vi "Fitz9 PID Control.vi"(7 "Pressure Controls":T2 {"output range"."output low" format="%.2f"; "output range"."output high" format="%.2f"; "PID gains"."derivative time (Td, min)" format="%.6f"; "PID gains"."integral time (Ti, min)" format="%.5f"; "PID gains"."proportional gain (Kc)" format="%.3f"; "Phi" scale=0.0..1.5; "Des P drop" scale=0.0..6.0}, 8 "Error In":errorcluster, 10 "Set Point Array":dbl[](array[numeric])) -> (0 "Error Out":errorcluster, 2 "Set Point Array out":dbl[](array[numeric]), 5 "Pressure Indicators":T1)   [LabVIEW 2013]
doc: "This sub-VI controls the air and fuel mass flow controllers for the Fitz9 burner. This burner has one air\nflow controller, and three fuel flow controllers, all with their own set points."
uses:
  Controls/pressure_control_cluster.ctl
  Controls/run_mode_enum.ctl
  Controls/Fitz9_pressure_indicator_cluster.ctl
  <vilib>/DAQmx/read.llb/DAQmx Read (Analog DBL 1Chan 1Samp).vi
  <vilib>/DAQmx/write.llb/DAQmx Write (Analog DBL 1Chan 1Samp).vi
  <vilib>/addons/control/pid/pid.llb/PID (DBL).vi
  <vilib>/DAQmx/miscellaneous.llb/DAQmx Fill In Error Info.vi
  <vilib>/addons/control/pid/NI_PID_pid.lvlib
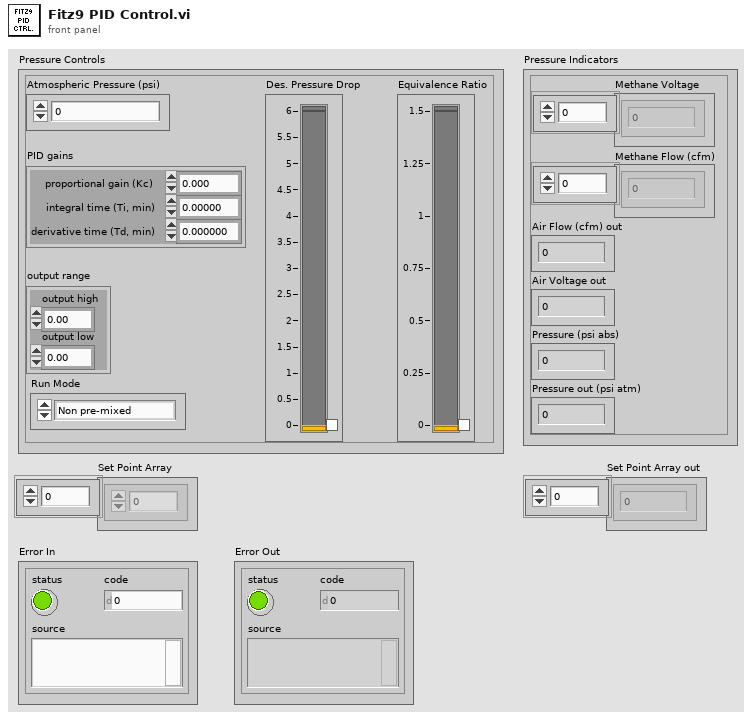
[diagram p1: front panel]
types:
  T1 = typedef "Fitz9_pressure_indicator_cluster.ctl" = cluster{"Methane Voltage":dbl[], "Methane Flow (cfm)":dbl[], "Air Flow (cfm) out":dbl, "Air Voltage out":dbl, "Pressure (psi abs)":dbl, "Pressure out (psi atm)":dbl}
  T2 = typedef "pressure_control_cluster.ctl" = cluster{"Atm Press":dbl, "Des P drop":dbl, "Phi":dbl, "PID gains":cluster{"proportional gain (Kc)":dbl, "integral time (Ti, min)":dbl, "derivative time (Td, min)":dbl}, "output range":cluster{"output high":dbl, "output low":dbl}, "Run Mode":T3}
  T3 = typedef "run_mode_enum.ctl" = enum16{"Non pre-mixed", "Pre-mixed"}
  T4 = cluster{"proportional gain (Kc)":dbl, "integral time (Ti, min)":dbl, "derivative time (Td, min)":dbl}
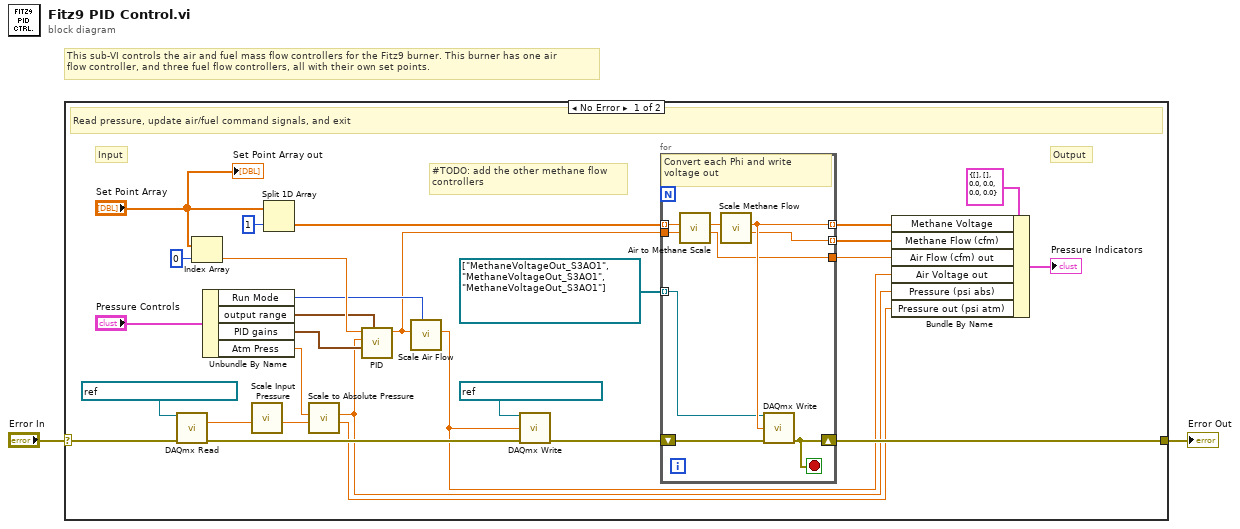
[diagram p0: block diagram]
diagram:
  # "This sub-VI controls the air and fuel mass flow controllers for the Fitz9 burner. This burner has one air\nflow controller, and three fuel flow controllers, all with their own set points."
  n1 = case shown="No Error" "Error In" {
    selector: "Error In" -> [w30 w40]
    tunnel: [w16 w40] -> w1
    frame No Error {
      # "Output"
      # "#TODO: add the other methane flow\ncontrollers"
      # "Input"
      # "Read pressure, update air/fuel command signals, and exit"
      n2 = call-poly <vilib>:"DAQmx Read.vi"("task/channels in"=refnum<k21> "PressureVoltageIn_S3AI8", "error in"=w30) -> ("data"=w27:dbl, "error out"=w29:errorcluster)  [unwired: 11 in, 1 out]
      n3 = Index Array(array="Set Point Array", index=0) -> (element=w24:dbl)
      n4 = Unbundle By Name("Pressure Controls") -> ("Run Mode"=w18:T3, "output range"=w21:cluster{"output high":dbl, "output low":dbl}, "PID gains"=w20:T4, "Atm Press"=w22:dbl)
      n5 = call "Scale Input Pressure.vi"("Pressure (V)"=w27) -> ("Pressure (psi atm)"=w26:dbl)  [unwired: 10 in]
      n6 = Split 1D Array(array="Set Point Array", index=1) -> (second subarray=w14:dbl[])  [unwired: 1 out]
      n7 = call "Scale to Absolute Pressure.vi"("Pressure (psi atm)"=w26, "Atm Press"=w22) -> ("Pressure out (psi atm)"=w4:dbl, "Pressure (psi abs)"=w5:dbl)  [unwired: 8 in]
      n8 = call-poly <vilib>:"PID.vi"("output range"=w21, "PID gains"=w20, "process variable"=w5, "setpoint"=w24) -> ("output"=w13:dbl)  [unwired: 6 in, 1 out]
      n9 = call "Scale Air Flow.vi"("Run Mode"=w18, "Air Flow (cfm)"=w13) -> ("Air Voltage out"=w6:dbl)  [unwired: 8 in, 1 out]
      n10 = call-poly <vilib>:"DAQmx Write.vi"("task/channels in"=refnum<k21> "AirVoltageOut_S3AO0", "data"=w6, "error in"=w29) -> ("error out"=w17:errorcluster)  [unwired: 10 in, 2 out]
      n11 = for {
        shift-right: [w35] -> w16
        shift-left: w17 -> [w39]
        tunnel: w14 -> [w37] mode=indexing
        tunnel: w13 -> [w36]
        tunnel: [w34] -> w9 mode=indexing
        tunnel: [w31] -> w8 mode=indexing
        tunnel: refnum<k21>[] ["MethaneVoltageOut_S3AO1", "MethaneVoltageOut_S3AO1", "MethaneVoltageOut_S3AO1"] -> [w33] mode=indexing
        tunnel: [w32] -> w7
        stop <- w35 stop-if-true
        # "Convert each Phi and write voltage out"
        n12 = call "Air to Methane Scale.vi"("Air Flow (cfm)"=w36, "Phi"=w37) -> ("Air Flow (cfm) out"=w32:dbl, "Methane Flow (cfm)"=w38:dbl)  [unwired: 8 in]
        n13 = call "Scale Methane Flow.vi"("Methane flow (cfm)"=w38) -> ("Methan Flow (cfm) out"=w31:dbl, "Methane Voltage out"=w34:dbl)  [unwired: 9 in]
        n14 = call-poly <vilib>:"DAQmx Write.vi"("task/channels in"=w33, "data"=w34, "error in"=w39) -> ("error out"=w35:errorcluster)  [unwired: 10 in, 2 out]
      }
      n15 = Bundle By Name(cluster=T1 {"Methane Voltage"=[], "Methane Flow (cfm)"=[], "Air Flow (cfm) out"=0.0, "Air Voltage out"=0.0, "Pressure (psi abs)"=0.0, "Pressure out (psi atm)"=0.0} ("Pressure Indicators 2"), "Methane Voltage"=w9, "Methane Flow (cfm)"=w8, "Air Flow (cfm) out"=w7, "Air Voltage out"=w6, "Pressure (psi abs)"=w5, "Pressure out (psi atm)"=w4) -> (→"Pressure Indicators":T1)
      "Set Point Array out" <- "Set Point Array"
    }
    frame Error {
      # "Pass through and exit"
    }
  }
  "Error Out" <- w1
